vi "ViscometerZeroFGV.vi"(3 "Enum":enum16{"Set RPM", "Set Zero", "Get Value"}(ring), 7 "Zero_write":dbl, 11 "RPM_write":dbl) -> (8 "Zero_read":dbl, 15 "RPM_read":dbl)   [LabVIEW 2019]
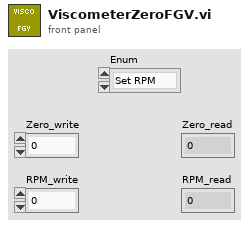
[diagram p1: front panel]
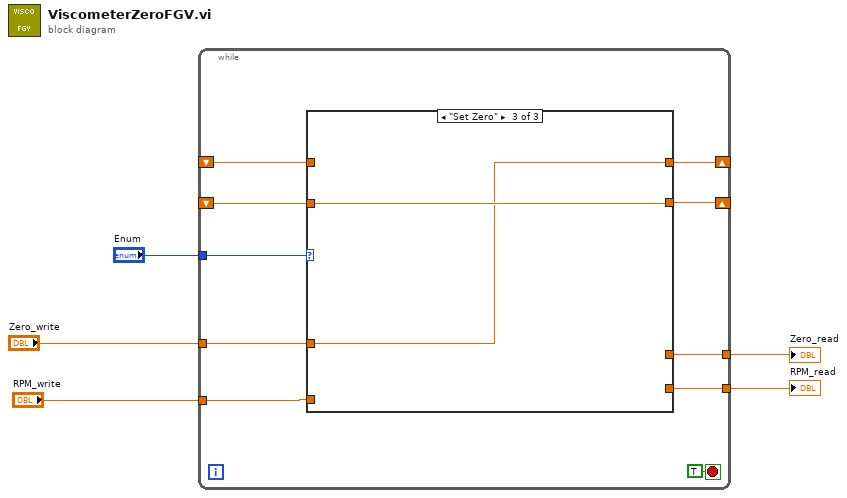
[diagram p0: block diagram]
diagram:
  n1 = while {
    tunnel: "Enum" -> [w15]
    shift-right: [w13] -> _
    shift-left: _ -> [w14]
    tunnel: [w12] -> w1
    tunnel: "Zero_write" -> [w10]
    tunnel: "RPM_write" -> [w9]
    shift-right: [w8] -> _
    shift-left: _ -> [w7]
    tunnel: [w6] -> w2
    stop <- TRUE ("stop") stop-if-true
    n2 = case shown="\"Set Zero\"" w15 {
      tunnel: w10 -> [_ _ w20]
      tunnel: w14 -> [w16 w19 _]
      tunnel: [w16 w19 w20] -> w13
      tunnel: [_ w19 _] -> w12
      tunnel: w9 -> [w17 _ _]
      tunnel: [w17 w18 w21] -> w8
      tunnel: w7 -> [_ w18 w21]
      tunnel: [_ w18 _] -> w6
      frame "Set RPM", Default {
      }
      frame "Get Value" {
      }
      frame "Set Zero" {
      }
    }
  }
  "Zero_read" <- w1
  "RPM_read" <- w2
